vi "toJSON.vi"(8 "error in (no error)":errorcluster, 11 "tBSONObjectID in":refnum<class "tBSONObjectID.lvclass">) -> (0 "error out":errorcluster, 2 "JSON":string, 3 "tBSONObjectID out":refnum<class "tBSONObjectID.lvclass">)   [LabVIEW 2013, in "BSON.lvlib" / "tBSONObjectID.lvclass"]
uses:
  tBSONObjectID.lvclass
  tBSONElement/tBSONElement.lvclass
  getValue.vi
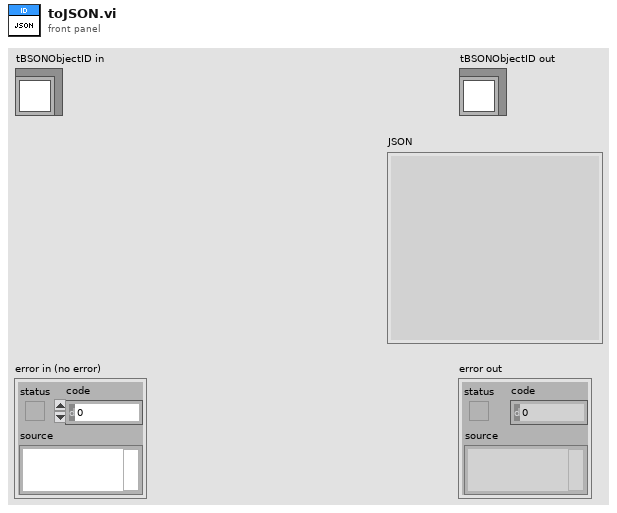
[diagram p1: front panel]
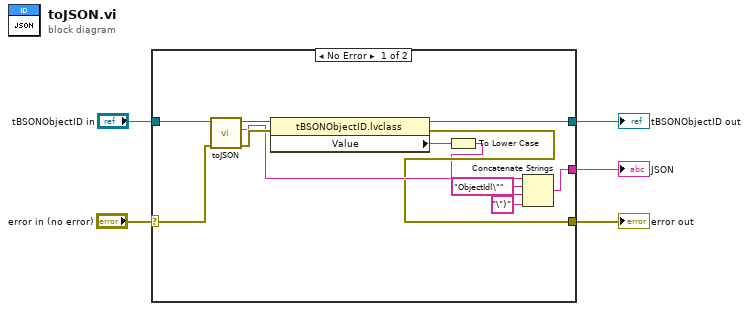
[diagram p0: block diagram]
diagram:
  n1 = case shown="No Error" "error in (no error)" {
    selector: "error in (no error)" -> [w14 w19]
    tunnel: "tBSONObjectID in" -> [w17 w18]
    tunnel: [w11 w19] -> w3
    tunnel: [w10 w18] -> w2
    tunnel: [w12 _] -> w1
    frame No Error {
      n2 = call-parent "toJSON.vi"("error in (no error)"=w14, "tBSONElement in"=w17) -> ("error out"=w15:errorcluster, "JSON"=w13:string, "tBSONElement out"=w16:refnum<class "tBSONObjectID.lvclass">)  [unwired: 7 in]
      n3 = property class="tBSONObjectID.lvclass"(reference=w16, error in=w15) -> (reference out=w10:refnum<class "tBSONObjectID.lvclass">, error out=w11:errorcluster, "Value"=w7:string)
      n4 = To Lower Case(string=w7) -> (all lower case string=w6:string)
      n5 = Concatenate Strings(w13, "ObjectId(\"" ("string"), w6, "\")" ("string")) -> (w12:string)
    }
    frame Error {
    }
  }
  "error out" <- w3
  "tBSONObjectID out" <- w2
  "JSON" <- w1
